vi "DFD Build MRate Filter.vi"   [LabVIEW 2017, in "NI_DigFilterLicensed.lvlib"]
doc: "Creates a multirate filter. You must manually select the polymorphic instance you want to use."
uses:
  <vilib>/addons/Digital Filter Design/NI_DigFilterLicensed.lvlib
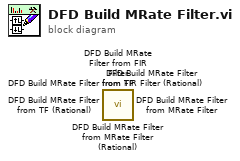
[diagram p0: block diagram]
diagram:
  n1 = call <vilib>:"DFD Build MRate Filter from MRate Filter (Rational).vi"() -> ()  [unwired: 10 in, 2 out]
  n2 = call <vilib>:"DFD Build MRate Filter from FIR Filter (Rational).vi"() -> ()  [unwired: 10 in, 2 out]
  n3 = call <vilib>:"DFD Build MRate Filter from TF (Rational).vi"() -> ()  [unwired: 10 in, 2 out]
  n4 = call <vilib>:"DFD Build MRate Filter from MRate Filter.vi"() -> ()  [unwired: 10 in, 2 out]
  n5 = call <vilib>:"DFD Build MRate Filter from TF.vi"() -> ()  [unwired: 10 in, 2 out]
  n6 = call <vilib>:"DFD Build MRate Filter from FIR Filter.vi"() -> ()  [unwired: 10 in, 2 out]
